vi "everest_adc_comp_trim_init.vi"(1 "CHB":dbl, 2 "error in (no error)":errorcluster, 3 "VISA resource name":refnum<visa-resource-name>="COM3") -> (0 "error out":errorcluster)   [LabVIEW 2015]
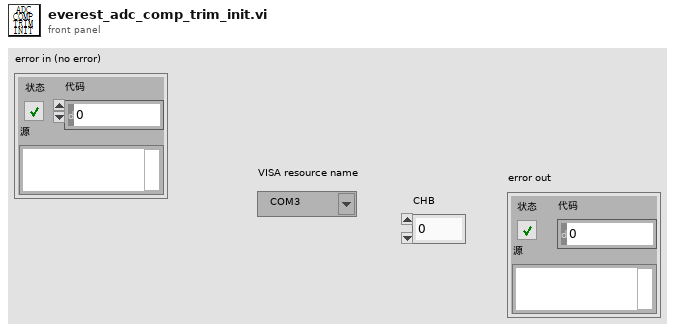
[diagram p1: front panel]
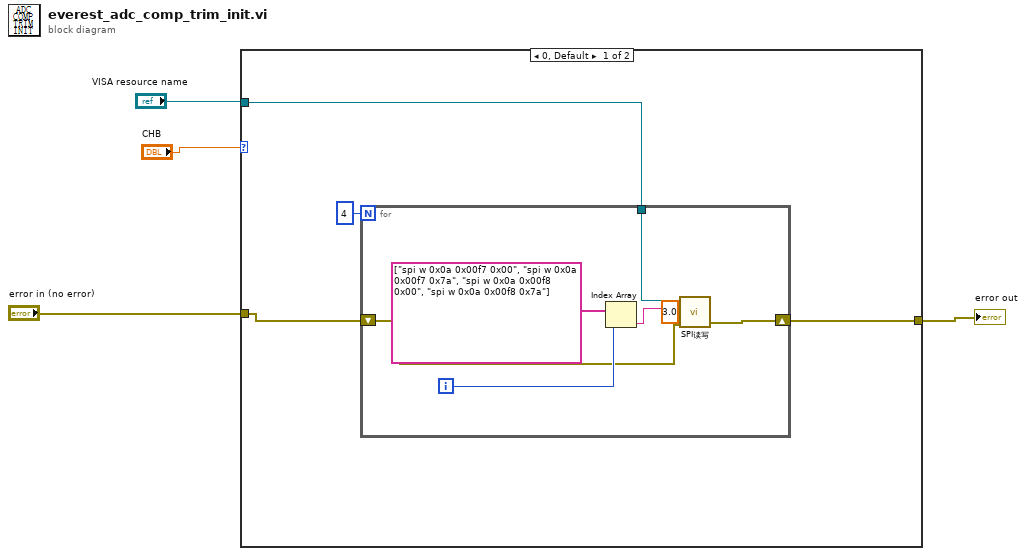
[diagram p0: block diagram]
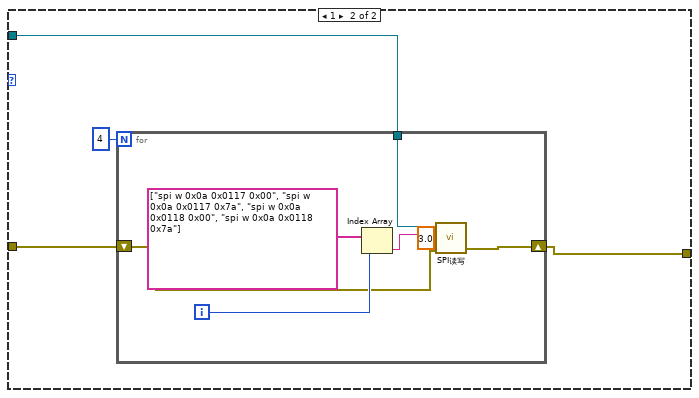
[diagram p2: hidden frame]
diagram:
  n1 = case shown="0, Default" "CHB" {
    tunnel: "error in (no error)" -> [w7 w17]
    tunnel: "VISA resource name" -> [w8 w19]
    tunnel: [w6 w16] -> w2
    frame 0, Default {
      n2 = for {
        N: 4 -> [_]
        tunnel: w8 -> [w12]
        shift-right: [w10] -> w6
        shift-left: w7 -> [w11]
        i -> [w14]
        n3 = Index Array(array=string[] ["spi w 0x0a 0x00f7 0x00", "spi w 0x0a 0x00f7 0x7a", "spi w 0x0a 0x00f8 0x00", "spi w 0x0a 0x00f8 0x7a"], index=w14) -> (element=w13:string)
        n4 = call "SPI读写.vi"("DELAY"=3.0, "error in (no error)"=w11, "往芯片写数据"=w13, "VISA resource name"=w12) -> ("error out"=w10:errorcluster)  [unwired: 1 in, 1 out]
      }
    }
    frame 1 {
      n5 = for {
        N: 4 -> [_]
        tunnel: w19 -> [w23]
        shift-right: [w21] -> w16
        shift-left: w17 -> [w22]
        i -> [w25]
        n6 = Index Array(array=string[] ["spi w 0x0a 0x0117 0x00", "spi w 0x0a 0x0117 0x7a", "spi w 0x0a 0x0118 0x00", "spi w 0x0a 0x0118 0x7a"], index=w25) -> (element=w24:string)
        n7 = call "SPI读写.vi"("DELAY"=3.0, "error in (no error)"=w22, "往芯片写数据"=w24, "VISA resource name"=w23) -> ("error out"=w21:errorcluster)  [unwired: 1 in, 1 out]
      }
    }
  }
  "error out" <- w2
